vi "Audio.Multi Tone Analysis.vi"(8 "Remove tones below FHz":dbl=500.0, 9 "max num tones":i32=4, 10 "threshold":dbl=0.001 format="%#_13g", 11 "Wvfrm In":waveform(dbl)(graph)={"t0"=timestamp(0 s since 1904-01-01), "dt"=2.2675736961451248e-05, "Y"=array[44100 elements]}) -> (1 "Tones":dbl[](array[numeric]) format="%.3f", 2 "multiple tone information":T2(array[cluster]) {"detected phase (deg)" format="%_6g"; "detected amplitude" format="%_6p"; "detected frequency" format="%_6p"}, 3 "Spectrum":T1(graph))   [LabVIEW 2018]
uses:
  <vilib>/measure/matone.llb/Extract Multiple Tone Information 1 Chan.vi
  <vilib>/measure/NI_MAPro.lvlib
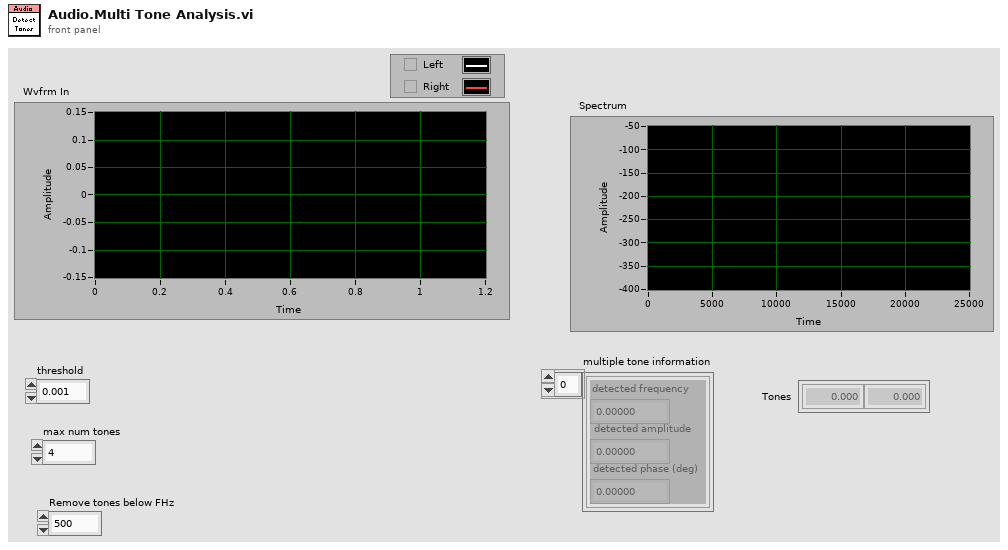
[diagram p1: front panel]
types:
  T1 = cluster{"f0":dbl, "df":dbl, "dB Spectrum (Hann)":dbl[]}
  T2 = cluster{"detected frequency":dbl, "detected amplitude":dbl, "detected phase (deg)":dbl}[]
  T3 = enum32{"none", "input signal", "detected signal", "residual signal"}
  T4 = cluster{"exported time signal":waveform(dbl), "exported spectrum (dB)":cluster{"f0":dbl, "df":dbl, "dB Spectrum (Hann)":dbl[]}}
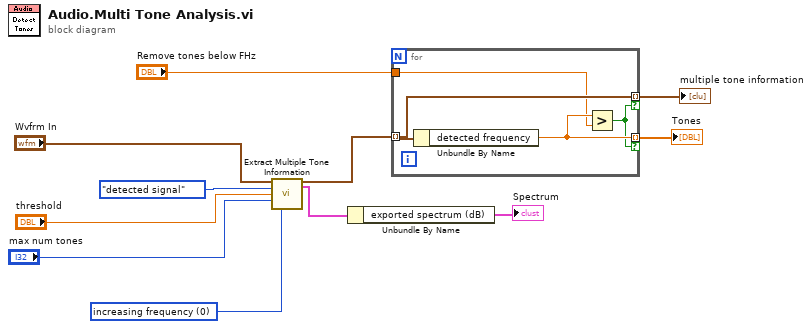
[diagram p0: block diagram]
diagram:
  w8 = 0 items=["increasing frequency", "decreasing amplitude"] ("output sorting")
  n1 = call-poly <vilib>:"Extract Multiple Tone Information.vi"("time signal in"="Wvfrm In", "export mode"=T3."detected signal", "threshold"="threshold", "max num tones"="max num tones", "output sorting"=w8) -> ("exported signals"=w6:T4, "multiple tone information"=w4:T2)  [unwired: 8 in, 1 out]
  n2 = Unbundle By Name(w6) -> ("exported spectrum (dB)"=→"Spectrum":T1)
  n3 = for {
    tunnel: w4 -> [w15] mode=indexing
    tunnel: [w14] -> w3 mode=indexing if=w12
    tunnel: [w15] -> w2 mode=indexing if=w12
    tunnel: "Remove tones below FHz" -> [w13]
    n4 = Unbundle By Name(w15) -> ("detected frequency"=w14:dbl)
    n5 = Greater?(x=w14, y=w13) -> (0:w12:bool)
  }
  "multiple tone information" <- w2
  "Tones" <- w3
